vi "set_value subroutine test.vi"() -> ()   [LabVIEW 2016]
uses:
  control vi/Beam Line Sections/R45.vi
  control vi/Beam Line Sections/R30.vi
  control vi/Beam Line Sections/Transmission.vi
  control vi/controls/beamline sections.lvlib
  control vi/R30/R30  library.lvlib
  control vi/Transmission/transmission.lvlib
panel:
  out "ControlsOnPage":refnum<vi>[](array[refnum])
  out "Array 3":string[](array[string])
  out "size(s)":i32
  out "Array 2":errorcluster[](array[cluster])
  out "error out":errorcluster
  out "Array":string[](array[string])
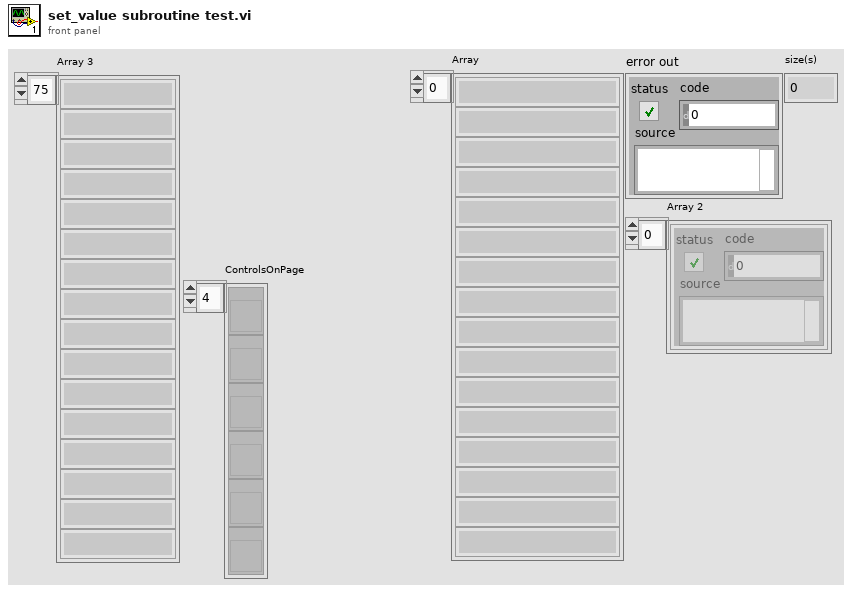
[diagram p1: front panel]
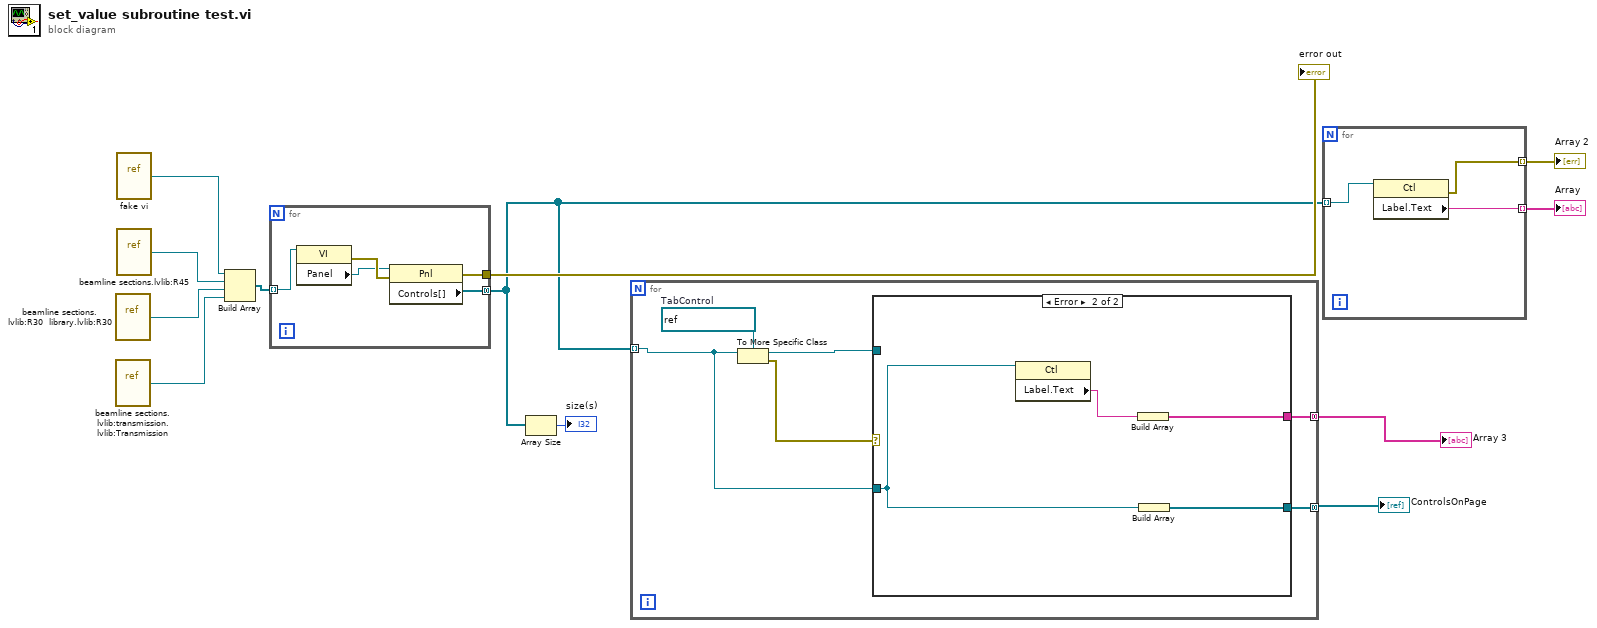
[diagram p0: block diagram]
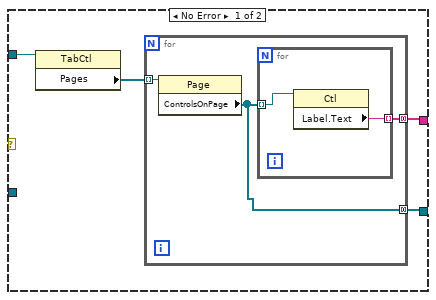
[diagram p2: hidden frame]
diagram:
  n1 = vi-ref "beamline sections.lvlib:R30  library.lvlib:R30.vi"() -> (w7:refnum<vi>)
  n2 = vi-ref "beamline sections.lvlib:transmission.lvlib:Transmission.vi"() -> (w8:refnum<vi>)
  n3 = vi-ref "fake vi.vi"() -> (w4:refnum<vi>)
  n4 = vi-ref "beamline sections.lvlib:R45.vi"() -> (w6:refnum<vi>)
  n5 = Build Array(w4, w6, w7, w8) -> (w5:refnum<vi>[])
  n6 = for {
    tunnel: [w15] -> w11
    tunnel: [w14] -> w3 mode=concatenating
    tunnel: w5 -> [w13] mode=indexing
    n7 = property class="VI"(reference=w13) -> (error out=w17:errorcluster, "Panel"=w16:refnum<vi>)  [unwired: 1 in, 1 out]
    n8 = property class="Pnl"(reference=w16, error in=w17) -> (error out=w15:errorcluster, "Controls[]"=w14:refnum<vi>[])  [unwired: 1 out]
  }
  "error out" <- w11
  n9 = Array Size(array=w3) -> (size(s)=→"size(s)":i32)
  n10 = for {
    tunnel: w3 -> [w18] mode=indexing
    tunnel: [w21] -> w2 mode=concatenating
    tunnel: [w20] -> w1 mode=concatenating
    w23 = refnum<vi> refnum  # TabControl
    n11 = To More Specific Class(target class=w23, reference=w18) -> (specific class reference=w22:refnum<vi>, error out=w19:errorcluster)  [unwired: 1 in]
    n12 = case shown="Error" w19 {
      tunnel: w22 -> [w27 _]
      tunnel: [w25 w34] -> w21
      tunnel: [w24 w33] -> w20
      tunnel: w18 -> [_ w36]
      frame No Error {
        n13 = property class="TabCtl"(reference=w27) -> ("Pages"=w26:refnum<vi>[])  [unwired: 1 in, 2 out]
        n14 = for {
          tunnel: w26 -> [w30] mode=indexing
          tunnel: [w29] -> w25 mode=concatenating
          tunnel: [w28] -> w24 mode=concatenating
          n15 = property class="Page"(reference=w30) -> ("ControlsOnPage"=w28:refnum<vi>[])  [unwired: 1 in, 2 out]
          n16 = for {
            tunnel: w28 -> [w32] mode=indexing
            tunnel: [w31] -> w29 mode=indexing
            n17 = property class="Ctl"(reference=w32) -> ("Label.Text"=w31:string)  [unwired: 1 in, 2 out]
          }
        }
      }
      frame Error {
        n18 = property class="Ctl"(reference=w36) -> ("Label.Text"=w35:string)  [unwired: 1 in, 2 out]
        n19 = Build Array(w35) -> (w34:string[])
        n20 = Build Array(w36) -> (w33:refnum<vi>[])
      }
    }
  }
  "Array 3" <- w2
  "ControlsOnPage" <- w1
  n21 = for {
    tunnel: w3 -> [w39] mode=indexing
    tunnel: [w38] -> w12 mode=indexing
    tunnel: [w37] -> w10 mode=indexing
    n22 = property class="Ctl"(reference=w39) -> (error out=w37:errorcluster, "Label.Text"=w38:string)  [unwired: 1 in, 1 out]
  }
  "Array" <- w12
  "Array 2" <- w10
